vi "Wavelength to Wavenumber.vi"(11 "Wavelength":dbl) -> (3 "Wavenumber":i32)   [LabVIEW 2018]
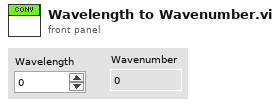
[diagram p1: front panel]
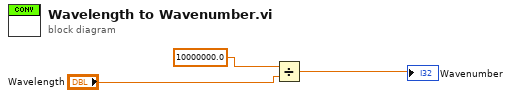
[diagram p0: block diagram]
diagram:
  n1 = Divide(x=10000000.0 ("y"), y="Wavelength") -> (x/y=→"Wavenumber":dbl)
